vi "ComputeFlagBits.vi"(8 "RETAIN":bool, 9 "QoS":T1, 10 "DUP":bool, 11 "Control Packet Type":T2) -> (3 "Flag Bits":u8 format="%04b")   [LabVIEW 2013]
uses:
  Control Packet Type -- enum.ctl
  QualityOfService -- enum.ctl
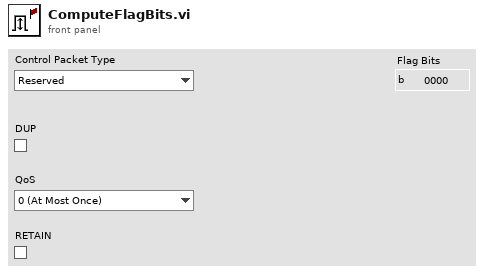
[diagram p1: front panel]
types:
  T1 = typedef "QualityOfService -- enum.ctl" = enum16{"0 (At Most Once)", "1 (At Least Once)", "2 (Exactly Once)"}
  T2 = typedef "Control Packet Type -- enum.ctl" = enum16{"Reserved", "CONNECT", "CONNACK", "PUBLISH", "PUBACK", "PUBREC", "PUBREL", "PUBCOMP", "SUBSCRIBE", "SUBACK", "UNSUBSCRIBE", "UNSUBACK", "PINGREQ", "PINGRESP", "DISCONNECT", "Reserved(15)"}
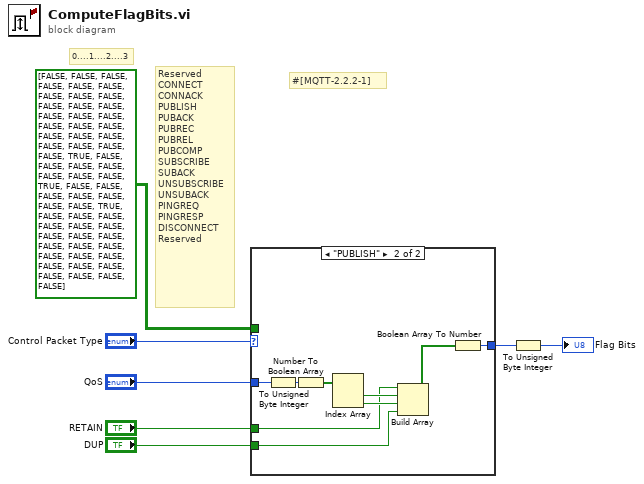
[diagram p0: block diagram]
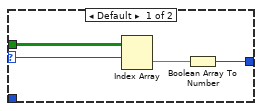
[diagram p2: hidden frame]
diagram:
  # "#[MQTT-2.2.2-1]"
  # "0....1....2....3"
  # "Reserved\nCONNECT\nCONNACK\nPUBLISH\nPUBACK\nPUBREC\nPUBREL\nPUBCOMP\nSUBSCRIBE\nSUBACK\nUNSUBSCRIBE\nUNSUBACK\nPINGREQ\nPINGRESP\nDISCONNECT\nReserved"
  n1 = case shown="\"PUBLISH\"" "Control Packet Type" {
    selector: "Control Packet Type" -> [w8 _]
    tunnel: [w11 w20] -> w7
    tunnel: bool[][] [[FALSE, FALSE, FALSE, FALSE], [FALSE, FALSE, FALSE, FALSE], [FALSE, FALSE, FALSE, FALSE], [FALSE, FALSE, FALSE, FALSE], [FALSE, FALSE, FALSE, FALSE], [FALSE, FALSE, FALSE, FALSE], [FALSE, TRUE, FALSE, FALSE], [FALSE, FALSE, FALSE, FALSE], [FALSE, TRUE, FALSE, FALSE], [FALSE, FALSE, FALSE, FALSE], [FALSE, TRUE, FALSE, FALSE], [FALSE, FALSE, FALSE, FALSE], [FALSE, FALSE, FALSE, FALSE], [FALSE, FALSE, FALSE, FALSE], [FALSE, FALSE, FALSE, FALSE], [FALSE, FALSE, FALSE, FALSE]] ("Boolean array") -> [w10 _]
    tunnel: "QoS" -> [_ w19]
    tunnel: "RETAIN" -> [_ w13]
    tunnel: "DUP" -> [_ w12]
    frame Default {
      n2 = Index Array(array=w10, index (row)=w8) -> (element=w9:bool[])  [unwired: 1 in]
      n3 = Boolean Array To Number(Boolean array=w9) -> (number=w11:u32)
    }
    frame "PUBLISH" {
      n4 = To Unsigned Byte Integer(number=w19) -> (unsigned 8bit integer=w18:u8)
      n5 = Number To Boolean Array(number=w18) -> (Boolean array=w16:bool[])
      n6 = Index Array(array=w16) -> (element #1=w15:bool, element #2=w14:bool)  [unwired: 2 in]
      n7 = Build Array(w13, w15, w14, w12) -> (w17:bool[])
      n8 = Boolean Array To Number(Boolean array=w17) -> (number=w20:u32)
    }
  }
  n9 = To Unsigned Byte Integer(number=w7) -> (unsigned 8bit integer=→"Flag Bits":u8)
